vi "Delegate Message.vi"(5 "Data":string, 7 "Stack ID":u8, 8 "error in (no error)":errorcluster, 10 "Function ID":u8, 11 "IP Connection in":refnum<class "IP Connection.lvclass">) -> (0 "error out":errorcluster, 3 "IP Connection out":refnum<class "IP Connection.lvclass">)   [LabVIEW 2011, in "Tinkerforge.lvlib" / "IP Connection.lvclass"]
doc: "This VI delegates non-global messages to the stack devices."
uses:
  IP Connection.lvclass
  Device/Device.lvclass
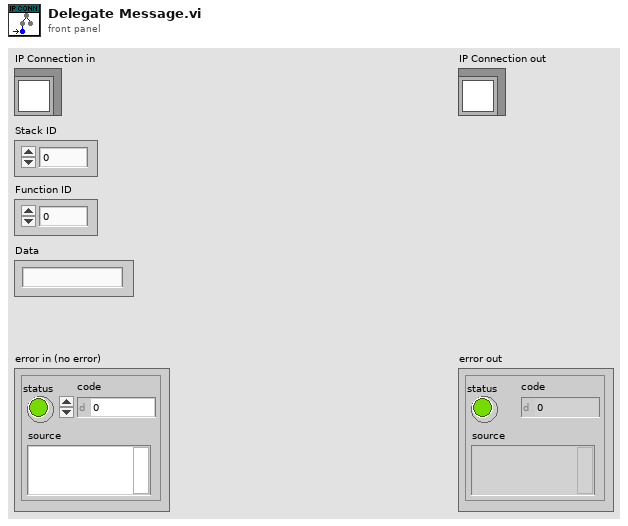
[diagram p1: front panel]
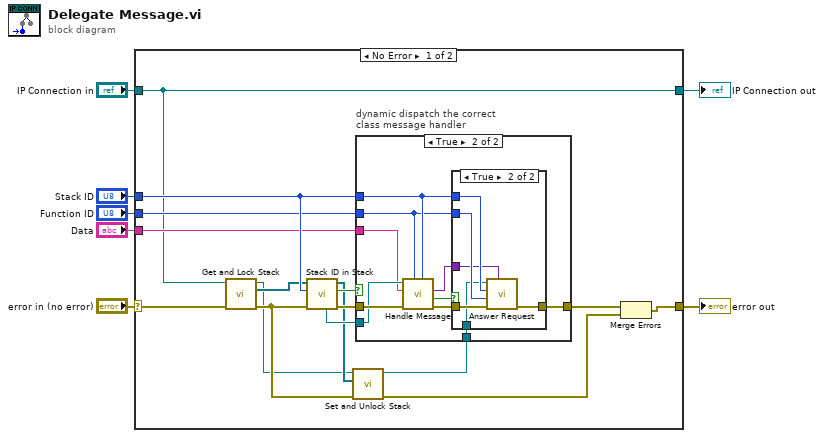
[diagram p0: block diagram]
diagram:
  n1 = case shown="No Error" "error in (no error)" {
    selector: "error in (no error)" -> [w15 w43]
    tunnel: [w23 w43] -> w6
    tunnel: [w14 w42] -> w4
    tunnel: "IP Connection in" -> [w14 w42]
    tunnel: "Stack ID" -> [w19 _]
    tunnel: "Function ID" -> [w18 _]
    tunnel: "Data" -> [w17 _]
    frame No Error {
      n2 = call "Get and Lock Stack.vi"("error in (no error)"=w15, "IP Connection in"=w14) -> ("error out"=w11:errorcluster, "Stack"=w13:refnum<class "Device.lvclass">[], "IP Connection out"=w9:refnum<class "IP Connection.lvclass">)  [unwired: 7 in]
      n3 = call "Stack ID in Stack.vi"("error in (no error)"=w11, "Stack ID"=w19, "Stack in"=w13) -> ("error out"=w22:errorcluster, "Device found?"=w21:bool, "Stack out"=w10:refnum<class "Device.lvclass">[], "Device out"=w20:refnum<class "Device.lvclass">)  [unwired: 4 in, 1 out]
      n4 = call "Set and Unlock Stack.vi"("error in (no error)"=w11, "Stack"=w10, "IP Connection in"=w9) -> ("error out"=w12:errorcluster, "IP Connection out"=w8:refnum<class "IP Connection.lvclass">)  [unwired: 7 in]
      n5 = case "dynamic dispatch the correct\nclass message handler" shown="True" w21 {
        tunnel: w22 -> [w24 w34]
        tunnel: w20 -> [_ w33]
        tunnel: w19 -> [_ w28]
        tunnel: w18 -> [_ w27]
        tunnel: w17 -> [_ w32]
        tunnel: [w24 w29] -> w16
        tunnel: w8 -> [_ w25]
        frame False {
        }
        frame True {
          n6 = call-dynamic "Handle Message.vi"("Stack ID"=w28, "Function ID"=w27, "error in (no error)"=w34, "Data"=w32, "Device in"=w33) -> ("error out"=w31:errorcluster, "Send Answer"=w30:bool, "Answer"=w26:variant)  [unwired: 3 in, 1 out]
          n7 = case shown="True" w30 {
            tunnel: w31 -> [w35 w41]
            tunnel: [w35 w40] -> w29
            tunnel: w28 -> [_ w39]
            tunnel: w27 -> [_ w38]
            tunnel: w26 -> [_ w37]
            tunnel: w25 -> [_ w36]
            frame False {
            }
            frame True {
              n8 = call "Answer Request.vi"("Data"=w37, "error in (no error)"=w41, "Function ID"=w38, "Stack ID"=w39, "IP Connection in"=w36) -> ("error out"=w40:errorcluster)  [unwired: 5 in, 1 out]
            }
          }
        }
      }
      n9 = Merge Errors(w16, w12) -> (w23:errorcluster)
    }
    frame Error {
    }
  }
  "error out" <- w6
  "IP Connection out" <- w4
